vi "Write_Stats_Impedance_Meas.vi"(4 "Z Phase":dbl[](array[numeric]), 5 "|Z| Mag":dbl[](array[numeric]), 6 "Output Stats Cluster":T1, 7 "Compensation and Gain":T2={"Rg_Vmon"=5000.0, "Rg_Imon"=5000.0, "ESL_Cal"=2.5e-07, "ESR_Cal"=0.0, "Cp_Cal"=0.0, "Rp_Cal"=0.0, "Use Open/Short\nCompensation"=FALSE, "R_Shunt"=10000.0}, 8 "Test Params Cluster":T3={"Test Freq. (Hz)"=0.0, "Output Signal Amplitude\nVolts Pk"=0.0, "Sampling Time (s)"=0.0, "Sampling Rate (Hz)"=0.0, "Output Channel"="Dev2/ao0", "Current Channel"="Dev2/ai0", "Voltage Channel"="Dev2/ai0", "Trigger Channel"="/Dev2/ao/StartTrigger", "Number of runs"=5}, 9 "Experiment Title":string="Experiment Title", 10 "File Name String":string="Test", 11 "Path":path=path "C:/Users/MPI/Documents/Test Saving Data") -> ()   [LabVIEW 2020]
panel:
  out "TDMS path":path=path "C:/Users/MPI/Documents/Test Saving Data/2022_01_06_23_07_06_Test.tdms"
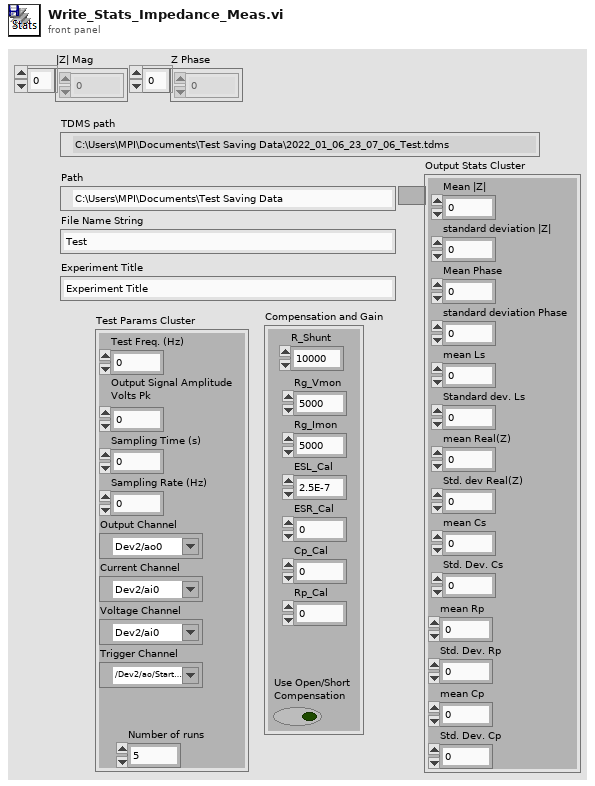
[diagram p1: front panel]
types:
  T1 = cluster{"Mean |Z|":dbl, "standard deviation |Z|":dbl, "Mean Phase":dbl, "standard deviation Phase":dbl, "mean Ls":dbl, "Standard dev. Ls":dbl, "mean Real(Z)":dbl, "Std. dev Real(Z)":dbl, "mean Cs":dbl, "Std. Dev. Cs":dbl, "Std. Dev. Rp":dbl, "mean Rp":dbl, "Std. Dev. Cp":dbl, "mean Cp":dbl}
  T2 = cluster{"Rg_Vmon":dbl, "Rg_Imon":dbl, "ESL_Cal":dbl, "ESR_Cal":dbl, "Cp_Cal":dbl, "Rp_Cal":dbl, "Use Open/Short\nCompensation":bool, "R_Shunt":dbl}
  T3 = cluster{"Test Freq. (Hz)":dbl, "Output Signal Amplitude\nVolts Pk":dbl, "Sampling Time (s)":dbl, "Sampling Rate (Hz)":dbl, "Output Channel":tag, "Current Channel":tag, "Voltage Channel":tag, "Trigger Channel":tag, "Number of runs":i32}
  T4 = enum16{"open", "open or create", "create or replace", "create", "open (read-only)"}
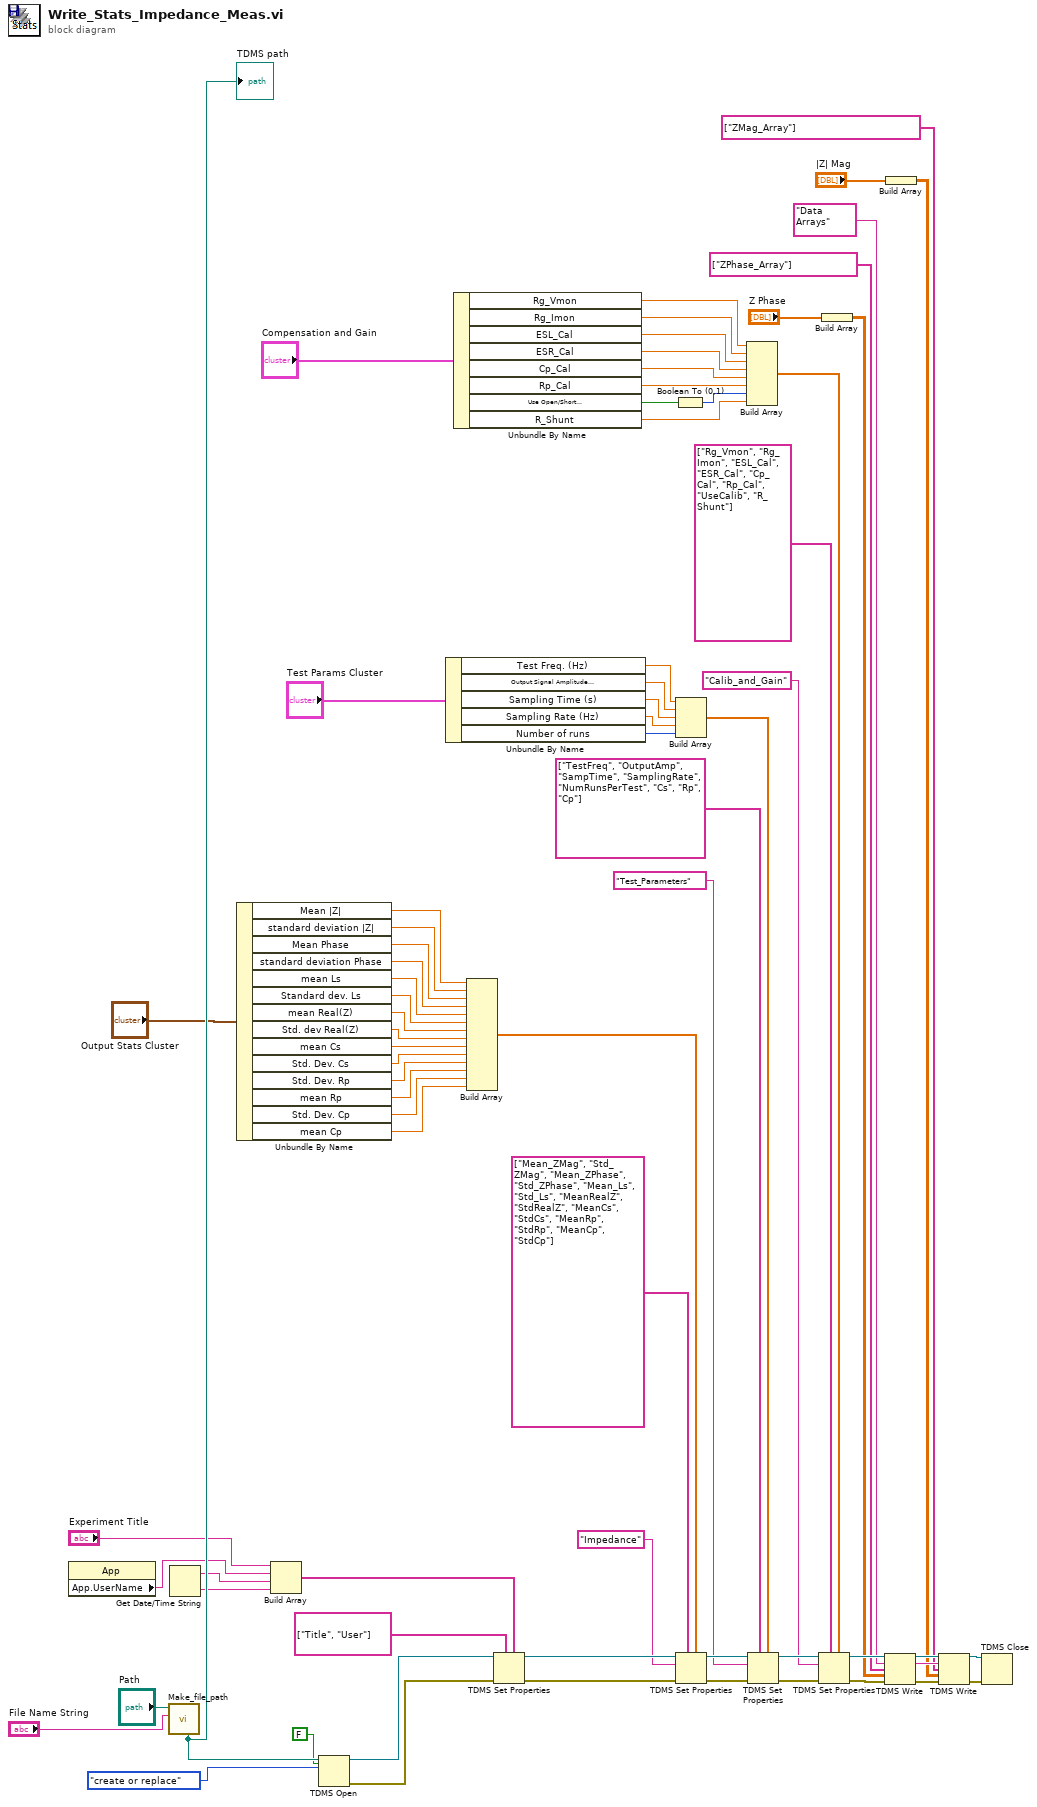
[diagram p0: block diagram]
diagram:
  n1 = property class="App"() -> ("App.UserName"=w68:string)  [unwired: 2 in, 2 out]
  n2 = call "Make_file_path.vi"("File Name String"="File Name String", "Base path"="Path") -> ("TDMS path"=w73:path)  [unwired: 9 in]
  "TDMS path" <- w73
  n3 = Get Date/Time String() -> (date string=w56:string, time string=w55:string)  [unwired: 3 in]
  n4 = Unbundle By Name("Output Stats Cluster") -> ("Mean |Z|"=w61:dbl, "standard deviation |Z|"=w59:dbl, "Mean Phase"=w58:dbl, "standard deviation Phase"=w57:dbl, "mean Ls"=w10:dbl, "Standard dev. Ls"=w9:dbl, "mean Real(Z)"=w8:dbl, "Std. dev Real(Z)"=w7:dbl, "mean Cs"=w6:dbl, "Std. Dev. Cs"=w5:dbl, "Std. Dev. Rp"=w4:dbl, "mean Rp"=w3:dbl, "Std. Dev. Cp"=w2:dbl, "mean Cp"=w1:dbl)
  n5 = Build Array("Experiment Title", w68, w56, w55) -> (w67:string[])
  n6 = TDMS Open(5:FALSE ("create index file? (T)"), 10:T4."create or replace" ("operation (0:open)"), 11:w73) -> (0:w25:errorcluster, 3:w65:refnum<k34>)  [unwired: 4 in]
  n7 = Unbundle By Name("Test Params Cluster") -> ("Test Freq. (Hz)"=w47:dbl, "Output Signal Amplitude\nVolts Pk"=w48:dbl, "Sampling Time (s)"=w49:dbl, "Sampling Rate (Hz)"=w50:dbl, "Number of runs"=w12:i32)
  n8 = Unbundle By Name("Compensation and Gain") -> ("Rg_Vmon"=w40:dbl, "Rg_Imon"=w39:dbl, "ESL_Cal"=w38:dbl, "ESR_Cal"=w37:dbl, "Cp_Cal"=w36:dbl, "Rp_Cal"=w35:dbl, "Use Open/Short\nCompensation"=w34:bool, "R_Shunt"=w31:dbl)
  n9 = Build Array(w61, w59, w58, w57, w10, w9, w8, w7, w6, w5, w4, w3, w2, w1) -> (w62:dbl[])
  n10 = TDMS Set Properties(5:w67, 7:string[] ["Title", "User"] ("property names"), 8:w25, 11:w65) -> (0:w24:errorcluster, 3:w64:refnum<k34>)  [unwired: 4 out]
  n11 = Boolean To (0,1)(Boolean=w34) -> (0, 1=w33:i16)
  n12 = Build Array(w47, w48, w49, w50, w12) -> (w46:dbl[])
  n13 = TDMS Set Properties(5:w62, 7:string[] ["Mean_ZMag", "Std_ZMag", "Mean_ZPhase", "Std_ZPhase", "Mean_Ls", "Std_Ls", "MeanRealZ", "StdRealZ", "MeanCs", "StdCs", "MeanRp", "StdRp", "MeanCp", "StdCp"] ("property names"), 8:w24, 10:"Impedance" ("group name"), 11:w64) -> (0:w23:errorcluster, 3:w52:refnum<k34>)  [unwired: 3 out]
  n14 = Build Array(w40, w39, w38, w37, w36, w35, w33, w31) -> (w32:dbl[])
  n15 = TDMS Set Properties(5:w46, 7:string[] ["TestFreq", "OutputAmp", "SampTime", "SamplingRate", "NumRunsPerTest", "Cs", "Rp", "Cp"] ("property names"), 8:w23, 10:"Test_Parameters" ("group name"), 11:w52) -> (0:w22:errorcluster, 3:w43:refnum<k34>)  [unwired: 3 out]
  n16 = TDMS Set Properties(5:w32, 7:string[] ["Rg_Vmon", "Rg_Imon", "ESL_Cal", "ESR_Cal", "Cp_Cal", "Rp_Cal", "UseCalib", "R_Shunt"] ("property names"), 8:w22, 10:"Calib_and_Gain" ("group name"), 11:w43) -> (0:w21:errorcluster, 3:w30:refnum<k34>)  [unwired: 3 out]
  n17 = Build Array("Z Phase") -> (w17:dbl[][])
  n18 = TDMS Write(0:w30, 5:"Data Arrays" ("group name"), 7:string[] ["ZPhase_Array"] ("channel name(s) in (Untitled)"), 9:w17, 11:w21) -> (4:w29:refnum<k34>, 6:w26:string, 15:w20:errorcluster)  [unwired: 1 in, 1 out]
  n19 = Build Array("|Z| Mag") -> (w15:dbl[][])
  n20 = TDMS Write(0:w29, 5:w26, 7:string[] ["ZMag_Array"] ("channel name(s) in (Untitled)"), 9:w15, 11:w20) -> (4:w28:refnum<k34>, 15:w19:errorcluster)  [unwired: 1 in, 2 out]
  n21 = TDMS Close(8:w19, 11:w28) -> ()  [unwired: 2 out]
